vi "Approach Target.vi"(4 "Indicator":refnum<vi>, 5 "Axial distance [um]":refnum<vi>, 8 "error in":errorcluster, 10 "Calibration":T1, 11 "Manipulator Interface":T2) -> (0 "error out":errorcluster, 2 "Error":bool)   [LabVIEW 2012, in "Targeting Unit.lvlib"]
uses:
  Targeting Unit.lvlib
  <vilib>/Analysis/Matrix/Datatypes/RealMatrix.ctl
  <vilib>/Analysis/Matrix/NI_Matrix.lvlib
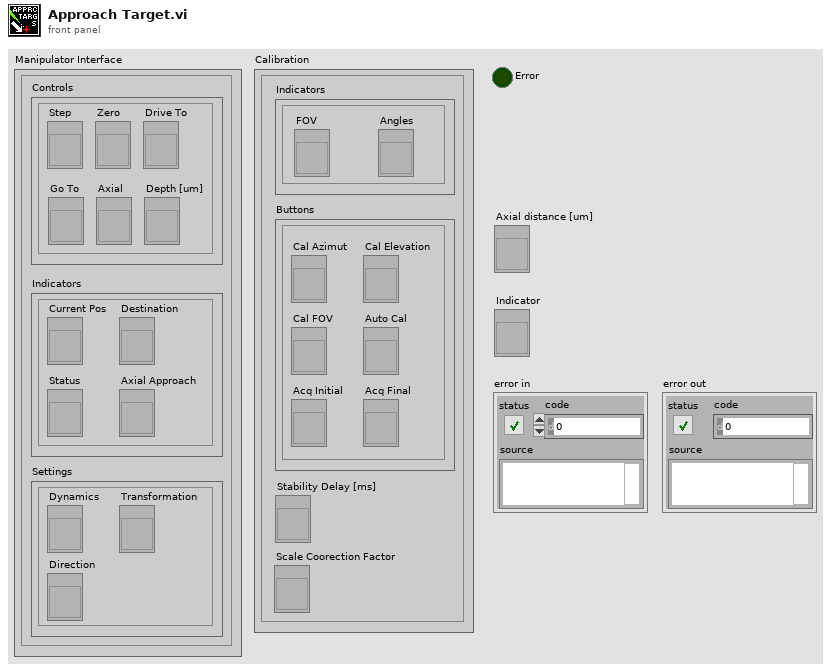
[diagram p1: front panel]
types:
  T1 = cluster{"Indicators":cluster{"FOV":refnum<vi>, "Angles":refnum<vi>}, "Buttons":cluster{"Cal FOV":refnum<vi>, "Cal Azimut":refnum<vi>, "Cal Elevation":refnum<vi>, "Auto Cal":refnum<vi>, "Acq Initial":refnum<vi>, "Acq Final":refnum<vi>}, "Stability Delay [ms]":refnum<vi>, "Scale Coorection Factor":refnum<vi>}
  T2 = cluster{"Indicators":cluster{"Current Pos":refnum<vi>, "Destination":refnum<vi>, "Status":refnum<vi>, "Axial Approach":refnum<vi>}, "Settings":cluster{"Dynamics":refnum<vi>, "Transformation":refnum<vi>, "Direction":refnum<vi>}, "Controls":cluster{"Zero":refnum<vi>, "Step":refnum<vi>, "Drive To":refnum<vi>, "Go To":refnum<vi>, "Axial":refnum<vi>, "Depth [um]":refnum<vi>}}
  T3 = cluster{"X [um]":dbl, "Y [um]":dbl, "Z [um]":dbl}
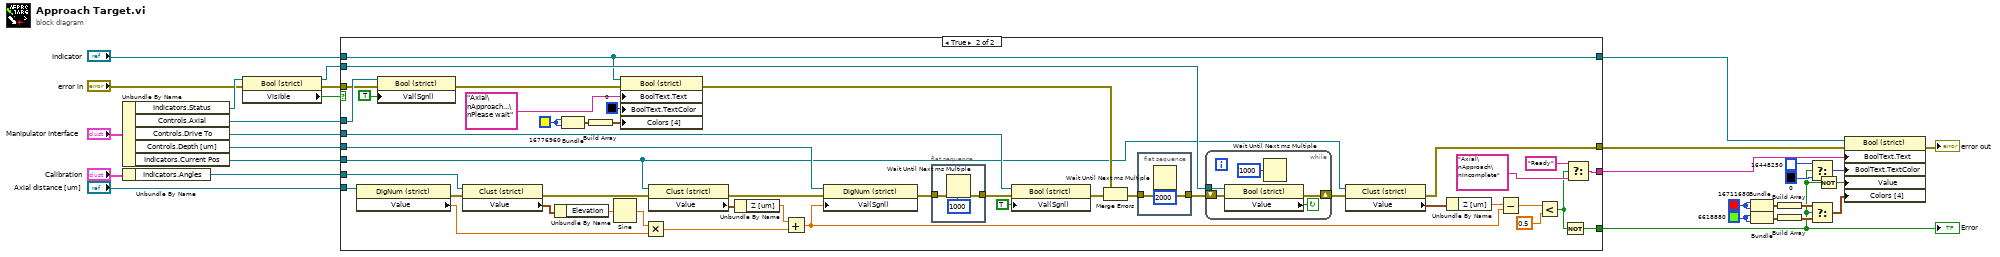
[diagram p0: block diagram]
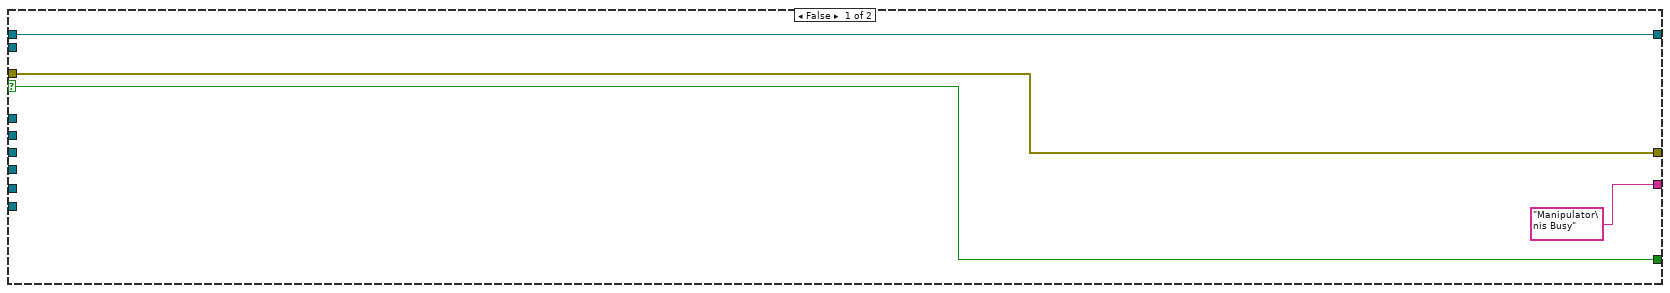
[diagram p2: hidden frame]
diagram:
  w18 = u32 6618880
  w15 = u32 16711680
  n1 = Unbundle By Name("Manipulator Interface") -> ("Indicators.Status"=w23:refnum<vi>, "Controls.Axial"=w24:refnum<vi>, "Controls.Drive To"=w27:refnum<vi>, "Controls.Depth [um]"=w28:refnum<vi>, "Indicators.Current Pos"=w5:refnum<vi>)
  n2 = Unbundle By Name("Calibration") -> ("Indicators.Angles"=w2:refnum<vi>)
  n3 = property class="Bool (strict)"(reference=w23, error in="error in") -> (reference out=w4:refnum<vi>, error out=w26:errorcluster, "Visible"=w29:bool)
  n4 = case shown="True" w29 {
    selector: w29 -> [w33 _]
    tunnel: w24 -> [_ w79]
    tunnel: w4 -> [_ w78]
    tunnel: w28 -> [_ w77]
    tunnel: w27 -> [_ w75]
    tunnel: ["Manipulator\nis Busy" ("Window Title (\"\")") w69] -> w8
    tunnel: [w33 w54] -> w7
    tunnel: w26 -> [w32 w66]
    tunnel: "Indicator" -> [w31 w58]
    tunnel: [w32 w59] -> w10
    tunnel: [w31 w58] -> w9
    tunnel: w5 -> [_ w35]
    tunnel: w2 -> [_ w44]
    tunnel: "Axial distance [um]" -> [_ w41]
    frame False {
    }
    frame True {
      w56 = u32 16776960
      n5 = property class="DigNum (strict)"(reference=w41) -> (error out=w39:errorcluster, "Value"=w40:dbl)  [unwired: 1 in, 1 out]
      n6 = property class="Bool (strict)"(reference=w79, error in=w66, "Val(Sgnl)"=TRUE ("Value")) -> (error out=w63:errorcluster)  [unwired: 1 out]
      n7 = property class="Clust (strict)"(reference=w44, error in=w39) -> (error out=w43:errorcluster, "Value"=w46:cluster{"Azimut":dbl, "Elevation":dbl})  [unwired: 1 out]
      n8 = Unbundle By Name(w46) -> ("Elevation"=w45:dbl)
      n9 = Bundle(w56, w56) -> (w57:cluster{u32, u32})  [unwired: 1 in]
      n10 = Build Array(w57) -> (w55:cluster{u32, u32}[])
      n11 = Sine(x=w45) -> (sin(x)=w42:dbl)
      n12 = property class="Bool (strict)"(reference=w58, error in=w63, "BoolText.Text"="Axial\nApproach...\nPlease wait" ("Window Title (\"\")"), "BoolText.TextColor"=u32 0, "Colors [4]"=w55) -> (error out=w60:errorcluster)  [unwired: 1 out]
      n13 = Multiply(x=w42, y=w40) -> (x*y=w38:dbl)
      n14 = property class="Clust (strict)"(reference=w35, error in=w43) -> (error out=w49:errorcluster, "Value"=w47:T3)  [unwired: 1 out]
      n15 = Unbundle By Name(w47) -> ("Z [um]"=w48:dbl)
      n16 = Add(x=w48, y=w38) -> (x+y=w50:dbl)
      n17 = property class="DigNum (strict)"(reference=w77, error in=w49, "Val(Sgnl)"=w50) -> (error out=w37:errorcluster)  [unwired: 1 out]
      n18 = flat-sequence {
        tunnel: w37 -> [w80]
        tunnel: [w80] -> w36
        frame #0 {
          n19 = Wait Until Next ms Multiple(millisecond multiple=u32 1000) -> ()  [unwired: 1 out]
        }
      }
      n20 = property class="Bool (strict)"(reference=w75, error in=w36, "Val(Sgnl)"=TRUE ("Value")) -> (error out=w61:errorcluster)  [unwired: 1 out]
      n21 = Merge Errors(w60, w61) -> (w52:errorcluster)
      n22 = flat-sequence {
        tunnel: [w83] -> w51
        tunnel: w52 -> [w83]
        frame #0 {
          n23 = Wait Until Next ms Multiple(millisecond multiple=u32 2000) -> ()  [unwired: 1 out]
        }
      }
      n24 = while {
        tunnel: w78 -> [w84]
        shift-right: [w85] -> w74
        shift-left: w51 -> [w86]
        stop <- w88 continue-if-true
        n25 = property class="Bool (strict)"(reference=w84, error in=w86) -> (error out=w85:errorcluster, "Value"=w88:bool)  [unwired: 1 out]
        n26 = Wait Until Next ms Multiple(millisecond multiple=u32 1000) -> ()  [unwired: 1 out]
      }
      n27 = property class="Clust (strict)"(reference=w35, error in=w74) -> (error out=w59:errorcluster, "Value"=w72:T3)  [unwired: 1 out]
      n28 = Unbundle By Name(w72) -> ("Z [um]"=w71:dbl)
      n29 = Subtract(x=w71, y=w50) -> (x-y=w73:dbl)
      n30 = Less?(x=w73, y=0.5) -> (x < y?=w53:bool)
      n31 = Not(x=w53) -> (.not. x?=w54:bool)
      n32 = Select(t="Ready", s=w53, f="Axial\nApproach\nIncomplete" ("t")) -> (s? t:f=w69:string)
    }
  }
  "Error" <- w7
  n33 = Bundle(w15, w15) -> (w16:cluster{u32, u32})  [unwired: 1 in]
  n34 = Bundle(w18, w18) -> (w19:cluster{u32, u32})  [unwired: 1 in]
  n35 = Build Array(w16) -> (w17:cluster{u32, u32}[])
  n36 = Build Array(w19) -> (w20:cluster{u32, u32}[])
  n37 = Select(t=u32 16448250, s=w7, f=u32 0) -> (s? t:f=w13:u32)
  n38 = Select(t=w17, s=w7, f=w20) -> (s? t:f=w21:cluster{u32, u32}[])
  n39 = Not(x=w7) -> (.not. x?=w14:bool)
  n40 = property class="Bool (strict)"(reference=w9, error in=w10, "BoolText.Text"=w8, "BoolText.TextColor"=w13, "Value"=w14, "Colors [4]"=w21) -> (error out=→"error out":errorcluster)  [unwired: 1 out]
